vi "Real A x B.vi"(2 "B":T1, 3 "A":T1) -> (0 "error":i32, 1 "A x B":T1)   [LabVIEW 2018, in "NI_AALBase.lvlib"]
doc: "Performs the multiplication of two input matrices or an input matrix and an input vector. The data types you wire to the <B>A</B> and <B>B</B> inputs determine the polymorphic instance to use."
uses:
  <vilib>/Analysis/NI_AALBase.lvlib
  RealMatrix.ctl
  <resource>/lvanlys.dll
  NI_Matrix.lvlib
panel:
  # "A x B"
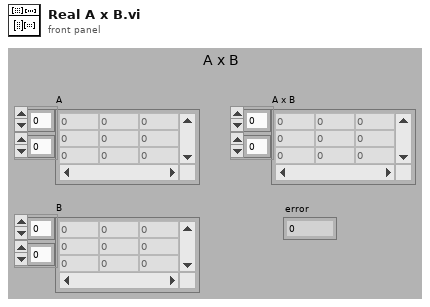
[diagram p1: front panel]
types:
  T1 = typedef "NI_Matrix.lvlib/RealMatrix.ctl" = dbl[][]
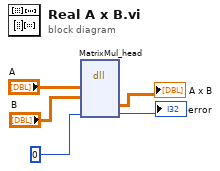
[diagram p0: block diagram]
diagram:
  n1 = dll-call lib="C:/Program Files (x86)/National Instruments/LabVIEW 2018/resource/lvanlys.*" fn="MatrixMul_head"("A"="A", "B"="B", 0) -> ("A x B"=→"A x B":T1, →"error":i32)  [unwired: 7 in, 2 out]
